vi "Access Privilege_Write Characters To File.vi"(0 "File path (dialog if empty)":path, 7 "Character string":string, 9 "Append to file? (new file:F)":bool, 10 "Convert eol? (no:F)":bool) -> (4 "new file path (Not A Path if cancelled)":path)   [LabVIEW 2023, in "GUI.lvlib"]
doc: "Writes a <B>character string</B> to a new byte stream file or appends the string to an existing file. The VI opens or creates the file before writing to it and closes it afterwards."
uses:
  GUI.lvlib
panel:
  in  "Prompt":string="Choose file to write."
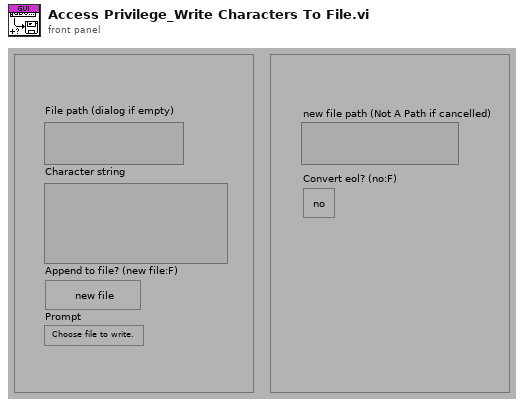
[diagram p1: front panel]
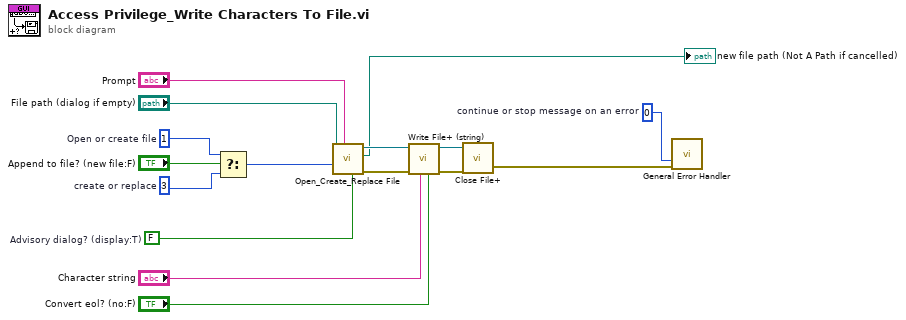
[diagram p0: block diagram]
diagram:
  w1 = FALSE  # Advisory dialog? (display:T)
  w8 = i16 3  # create or replace
  w14 = 0  # continue or stop message on an error
  w11 = i16 1  # Open or create file
  n1 = Select(t=w11, s="Append to file? (new file:F)", f=w8) -> (s? t:f=w3:i16)
  n2 = call <vilib>:"Open_Create_Replace File.vi"("advisory dialog? (display:T)"=w1, "prompt"="Prompt", "function (open:0)"=w3, "file path"="File path (dialog if empty)") -> ("error out"=w15:errorcluster, "new file path"=→"new file path (Not A Path if cancelled)":path, "refnum"=w7:refnum<file>)  [unwired: 3 in, 2 out]
  n3 = call <vilib>:"Write File+ (string).vi"("convert eol? (no:F)"="Convert eol? (no:F)", "string"="Character string", "error in (no error)"=w15, "refnum"=w7) -> ("error out"=w13:errorcluster, "dup refnum"=w12:refnum<file>)  [unwired: 2 in, 2 out]
  n4 = call <vilib>:"Close File+.vi"("error in (no error)"=w13, "refnum"=w12) -> ("error out"=w2:errorcluster)  [unwired: 5 out]
  n5 = call <vilib>:"General Error Handler.vi"("type of dialog (OK msg:1)"=w14, "error in (no error)"=w2) -> ()  [unwired: 1 in, 13 out]
